vi "Teleop.vi"(8 "Begin Cluster":T1={"Left Drive Encoder"={"DevStatus"={"status"=FALSE, "code"=0, "source"=""}, "EncoderIndex"=enum."Invalid", "CounterIndex"=enum."Ctr 1", "DistancePerCount"=2.0, "Decoding Type"=enum."4x"}, "Right Drive Encoder"={"DevStatus"={"status"=FALSE, "code"=0, "source"=""}, "EncoderIndex"=enum."Invalid", "CounterIndex"=enum."Ctr 1", "DistancePerCount"=2.0, "Decoding Type"=enum."4x"}, "Elevator Encoder"={"DevStatus"={"status"=FALSE, "code"=0, "source"=""}, "EncoderIndex"=enum."Invalid", "CounterIndex"=enum."Ctr 1", "DistancePerCount"=2.0, "Decoding Type"=enum."4x"}, "Drive Shifter"={"DevStatus"={"status"=FALSE, "code"=0, "source"=""}, "Pneumatics Control Module"=0, "Forward Solenoid Channel"=enum."Invalid", "Reverse Solenoid Channel"=enum."Invalid"}, "Elevator Shifter"={"DevStatus"={"status"=FALSE, "code"=0, "source"=""}, "Pneumatics Control Module"=0, "Forward Solenoid Channel"=enum."Invalid", "Reverse Solenoid Channel"=enum."Invalid"}, "Elevator Brake"={"DevStatus"={"status"=FALSE, "code"=0, "source"=""}, "Pneumatics Control Module"=0, "Forward Solenoid Channel"=enum."Invalid", "Reverse Solenoid Channel"=enum."Invalid"}, "Intake Clamp"={"DevStatus"={"status"=FALSE, "code"=0, "source"=""}, "Pneumatics Control Module"=0, "Forward Solenoid Channel"=enum."Invalid", "Reverse Solenoid Channel"=enum."Invalid"}, "Intake Hinge"={"DevStatus"={"status"=FALSE, "code"=0, "source"=""}, "Pneumatics Control Module"=0, "Forward Solenoid Channel"=enum."Invalid", "Reverse Solenoid Channel"=enum."Invalid"}, "Pot Left"={"DevStatus"={"status"=FALSE, "code"=0, "source"=""}, "Analog Channel"=enum."Invalid", "Invert Output"=FALSE}, "Pot Right"={"DevStatus"={"status"=FALSE, "code"=0, "source"=""}, "Analog Channel"=enum."Invalid", "Invert Output"=FALSE}, "Gyro"={"DevStatus"={"status"=FALSE, "code"=0, "source"=""}, "Analog Channel"=enum."AI 1", "Gain (VoltsPerDegree/Second)"=0.0, "Gyro Type"=enum."Analog", "Handle"=0, "SPI Bus"=enum."Invalid", "Device Found"=FALSE, "Sample Rate"=1.0, "Calibrate On Open"=FALSE, "Offset"=0.0}, "Drive Motors"={"DevStatus"={"status"=FALSE, "code"=0, "source"=""}, "Motors[]"=[], "Square Inputs"=FALSE, "Max Output"=1.0}, "Elevator Master"={"DeviceStatus"={"status"=FALSE, "code"=0, "source"=""}, "Type"=enum."PWM", "PWM"={"PWM Channel"=enum."Invalid", "DeadBand"={"Name"="", "maxPositivePwm"=0, "minPositivePwm"=0, "centerPwm"=0, "maxNegativePwm"=0, "minNegativePwm"=0, "angularRange"=0}}, "CAN"={"Device Number"=0, "SetOutput VI Ref"=variant(refnum<vi> refnum), "GetOutput VI Ref"=variant(refnum<vi> refnum), "Enable VI Ref"=variant(refnum<vi> refnum), "Disable VI Ref"=variant(refnum<vi> refnum), "Data"=variant}, "Invert"=FALSE, "DIO PWM"={"PWM \"Enable\" Channel"=enum."Invalid", "DIOChannel"=enum."Invalid", "PWM Rate"=0.0}}, "Intake Left"={"DeviceStatus"={"status"=FALSE, "code"=0, "source"=""}, "Type"=enum."PWM", "PWM"={"PWM Channel"=enum."Invalid", "DeadBand"={"Name"="", "maxPositivePwm"=0, "minPositivePwm"=0, "centerPwm"=0, "maxNegativePwm"=0, "minNegativePwm"=0, "angularRange"=0}}, "CAN"={"Device Number"=0, "SetOutput VI Ref"=variant(refnum<vi> refnum), "GetOutput VI Ref"=variant(refnum<vi> refnum), "Enable VI Ref"=variant(refnum<vi> refnum), "Disable VI Ref"=variant(refnum<vi> refnum), "Data"=variant}, "Invert"=FALSE, "DIO PWM"={"PWM \"Enable\" Channel"=enum."Invalid", "DIOChannel"=enum."Invalid", "PWM Rate"=0.0}}, "Intake Right"={"DeviceStatus"={"status"=FALSE, "code"=0, "source"=""}, "Type"=enum."PWM", "PWM"={"PWM Channel"=enum."Invalid", "DeadBand"={"Name"="", "maxPositivePwm"=0, "minPositivePwm"=0, "centerPwm"=0, "maxNegativePwm"=0, "minNegativePwm"=0, "angularRange"=0}}, "CAN"={"Device Number"=0, "SetOutput VI Ref"=variant(refnum<vi> refnum), "GetOutput VI Ref"=variant(refnum<vi> refnum), "Enable VI Ref"=variant(refnum<vi> refnum), "Disable VI Ref"=variant(refnum<vi> refnum), "Data"=variant}, "Invert"=FALSE, "DIO PWM"={"PWM \"Enable\" Channel"=enum."Invalid", "DIOChannel"=enum."Invalid", "PWM Rate"=0.0}}, "Linear Actuator Left"={"DeviceStatus"={"status"=FALSE, "code"=0, "source"=""}, "Type"=enum."PWM", "PWM"={"PWM Channel"=enum."Invalid", "DeadBand"={"Name"="", "maxPositivePwm"=0, "minPositivePwm"=0, "centerPwm"=0, "maxNegativePwm"=0, "minNegativePwm"=0, "angularRange"=0}}, "CAN"={"Device Number"=0, "SetOutput VI Ref"=variant(refnum<vi> refnum), "GetOutput VI Ref"=variant(refnum<vi> refnum), "Enable VI Ref"=variant(refnum<vi> refnum), "Disable VI Ref"=variant(refnum<vi> refnum), "Data"=variant}, "Invert"=FALSE, "DIO PWM"={"PWM \"Enable\" Channel"=enum."Invalid", "DIOChannel"=enum."Invalid", "PWM Rate"=0.0}}, "Linear Actuator Right"={"DeviceStatus"={"status"=FALSE, "code"=0, "source"=""}, "Type"=enum."PWM", "PWM"={"PWM Channel"=enum."Invalid", "DeadBand"={"Name"="", "maxPositivePwm"=0, "minPositivePwm"=0, "centerPwm"=0, "maxNegativePwm"=0, "minNegativePwm"=0, "angularRange"=0}}, "CAN"={"Device Number"=0, "SetOutput VI Ref"=variant(refnum<vi> refnum), "GetOutput VI Ref"=variant(refnum<vi> refnum), "Enable VI Ref"=variant(refnum<vi> refnum), "Disable VI Ref"=variant(refnum<vi> refnum), "Data"=variant}, "Invert"=FALSE, "DIO PWM"={"PWM \"Enable\" Channel"=enum."Invalid", "DIOChannel"=enum."Invalid", "PWM Rate"=0.0}}, "X Joystick"={"Device"=enum."USB 1"}, "Y Joystick"={"Device"=enum."USB 1"}, "Controller"={"Device"=enum."USB 1"}, "775 Drive Motors"={"DevStatus"={"status"=FALSE, "code"=0, "source"=""}, "Motors[]"=[], "Square Inputs"=FALSE, "Max Output"=1.0}, "Intake Angle Encoder"={"DevStatus"={"status"=FALSE, "code"=0, "source"=""}, "EncoderIndex"=enum."Invalid", "CounterIndex"=enum."Ctr 1", "DistancePerCount"=2.0, "Decoding Type"=enum."4x"}, "Intake Angle"={"DeviceStatus"={"status"=FALSE, "code"=0, "source"=""}, "Type"=enum."PWM", "PWM"={"PWM Channel"=enum."Invalid", "DeadBand"={"Name"="", "maxPositivePwm"=0, "minPositivePwm"=0, "centerPwm"=0, "maxNegativePwm"=0, "minNegativePwm"=0, "angularRange"=0}}, "CAN"={"Device Number"=0, "SetOutput VI Ref"=variant(refnum<vi> refnum), "GetOutput VI Ref"=variant(refnum<vi> refnum), "Enable VI Ref"=variant(refnum<vi> refnum), "Disable VI Ref"=variant(refnum<vi> refnum), "Data"=variant}, "Invert"=FALSE, "DIO PWM"={"PWM \"Enable\" Channel"=enum."Invalid", "DIOChannel"=enum."Invalid", "PWM Rate"=0.0}}} {"Gyro"."Sample Rate" min=0.25 max=100.0 step=0.25}, 10 "Match Info":T20={"Autonomous Elapsed Seconds"=0.0, "TeleOp Elapsed Seconds"=0.0, "Disabled Elapsed Seconds"=0.0, "Visited Autonomous"=FALSE, "Visited TeleOp"=FALSE, "Visited Disabled"=FALSE, "Autonomous Settings"={"Autonomous Style"=enum."Independent", "VI Refnum"=refnum}}, 11 "Call Context":T21) -> ()   [LabVIEW 2017]
doc: "This VI is called for each TeleOp packet received from the DS where the robot is not disabled. It is often used to read from the joysticks and update I/O or to update setpoints for timed control loops. It should complete and return within 20 milliseconds or it may miss DS packets."
uses:
  <vilib>/Rock Robotics/WPI/DriverStation/WPI_DriverStationDerivedRobotMode.ctl
  <vilib>/Rock Robotics/WPI/DriverStation/WPI_DriverStationMatch Info.ctl
  Begin Cluster.ctl
  <vilib>/Rock Robotics/WPI/Encoder/WPI_EncoderDevRef.ctl
  <vilib>/Rock Robotics/SystemInterfaces/Encoder/FPGA_EncoderIdx.ctl
  <vilib>/Rock Robotics/SystemInterfaces/Counter/FPGA_CounterCtrSystemIndex.ctl
  <vilib>/Rock Robotics/WPI/Encoder/WPI_EncoderType.ctl
  <vilib>/Rock Robotics/WPI/Solenoid/WPI_SolenoidDevRef.ctl
  <vilib>/Rock Robotics/WPI/Solenoid/WPI_SolenoidChannel.ctl
  <vilib>/Rock Robotics/WPI/Potentiometer/WPI_PotentiometerDevRef.ctl
  <vilib>/Rock Robotics/SystemInterfaces/AI/FPGA_AIChannel.ctl
  <vilib>/Rock Robotics/WPI/Gyro/WPI_GyroDevRef.ctl
  <vilib>/Rock Robotics/SystemInterfaces/spilib/spi_bus.ctl
  <vilib>/Rock Robotics/WPI/RobotDrive/WPI_RobotDriveDevRef.ctl
  <vilib>/Rock Robotics/WPI/MotorControl/WPI_MotorControlDeviceRef.ctl
  <vilib>/Rock Robotics/WPI/MotorControl/WPI_MotorControlType.ctl
  <vilib>/Rock Robotics/SystemInterfaces/DIO/FPGA_DIOPWMChannel.ctl
  <vilib>/Rock Robotics/WPI/PWM/WPI_PWMDeadband.ctl
  <vilib>/Rock Robotics/SystemInterfaces/DIO/FPGA_DIOChannel.ctl
  <vilib>/Rock Robotics/WPI/Joystick/WPI_JoystickDevRef.ctl
  <vilib>/Rock Robotics/WPI/Joystick/WPI_JoystickDeviceEnum.ctl
  <vilib>/Rock Robotics/WPI/RobotDrive/WPI_RobotDriveArcadeDrive_Standard(NoSaturation).vi
  Global Variables.vi
panel:
  in  "Drive State":bool
  in  "Elevator State":bool
  # "Analog"
  # "XRS"
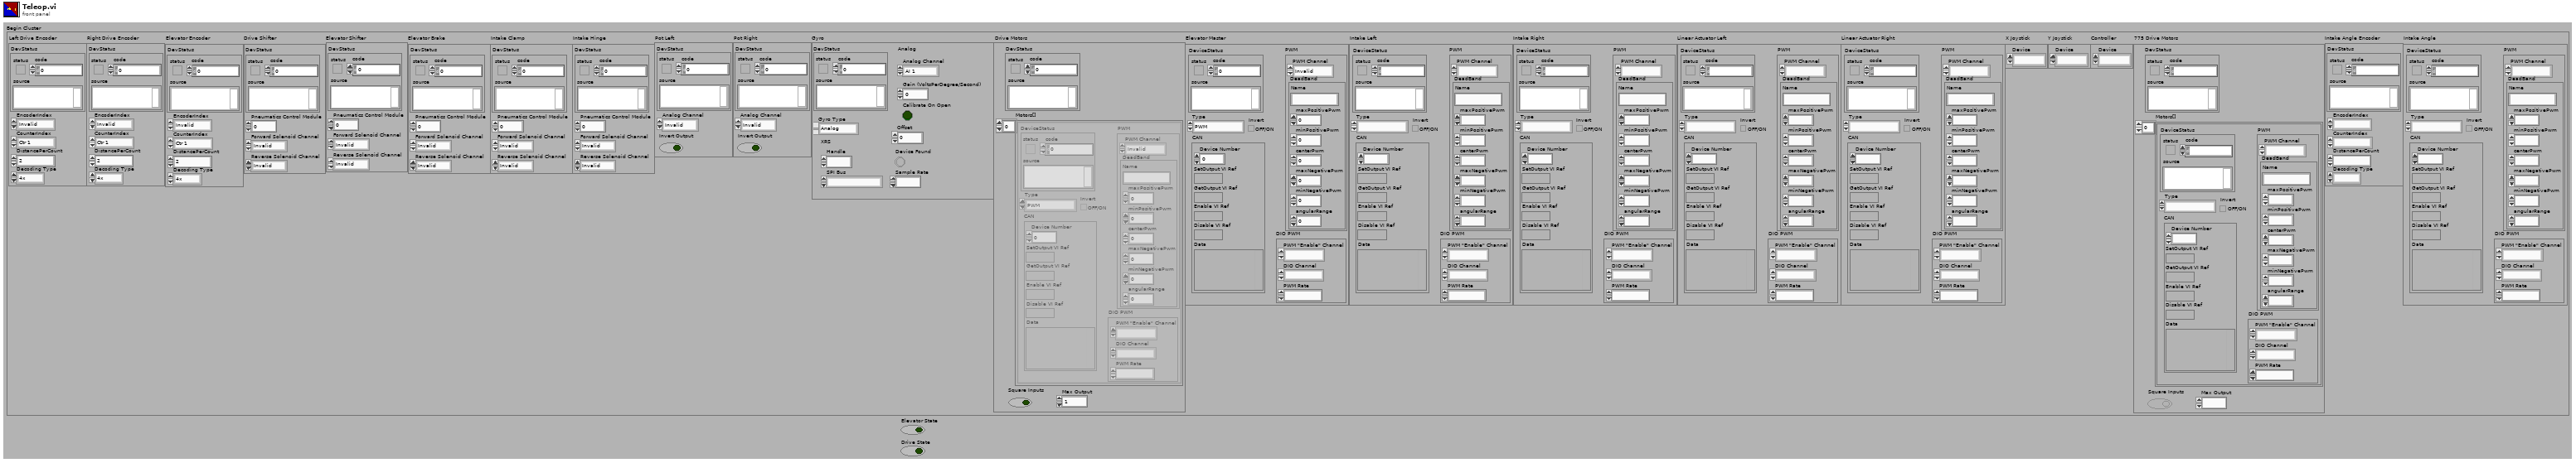
[diagram p1: front panel]
types:
  T1 = typedef "Begin Cluster.ctl" = cluster{"Left Drive Encoder":T2, "Right Drive Encoder":T2, "Elevator Encoder":T2, "Drive Shifter":T6, "Elevator Shifter":T6, "Elevator Brake":T6, "Intake Clamp":T6, "Intake Hinge":T6, "Pot Left":T8, "Pot Right":T8, "Gyro":T10, "Drive Motors":T12, "Elevator Master":T13, "Intake Left":T13, "Intake Right":T13, "Linear Actuator Left":T13, "Linear Actuator Right":T13, "X Joystick":T18, "Y Joystick":T18, "Controller":T18, "775 Drive Motors":T12, "Intake Angle Encoder":T2, "Intake Angle":T13}
  T2 = typedef "WPI_EncoderDevRef.ctl" = cluster{"DevStatus":errorcluster, "EncoderIndex":T3, "CounterIndex":T4, "DistancePerCount":dbl, "Decoding Type":T5}
  T3 = typedef "FPGA_EncoderIdx.ctl" = enum8{"Enc 0", "Enc 1", "Enc 2", "Enc 3", "Enc 4", "Enc 5", "Enc 6", "Enc 7", "Invalid"}
  T4 = typedef "FPGA_CounterCtrSystemIndex.ctl" = enum8{"Ctr 0", "Ctr 1", "Ctr 2", "Ctr 3", "Ctr 4", "Ctr 5", "Ctr 6", "Ctr 7", "Invalid"}
  T5 = typedef "WPI_EncoderType.ctl" = enum16{"1x", "2x", "4x"}
  T6 = typedef "WPI_SolenoidDevRef.ctl" = cluster{"DevStatus":errorcluster, "Pneumatics Control Module":u8, "Forward Solenoid Channel":T7, "Reverse Solenoid Channel":T7}
  T7 = typedef "WPI_SolenoidChannel.ctl" = enum8{"Solenoid 0", "Solenoid 1", "Solenoid 2", "Solenoid 3", "Solenoid 4", "Solenoid 5", "Solenoid 6", "Solenoid 7", "Invalid"}
  T8 = typedef "WPI_PotentiometerDevRef.ctl" = cluster{"DevStatus":errorcluster, "Analog Channel":T9, "Invert Output":bool}
  T9 = typedef "FPGA_AIChannel.ctl" = enum8{"AI 0", "AI 1", "AI 2", "AI 3", "AI MXP 0", "AI MXP 1", "AI MXP 2", "AI MXP 3", "Invalid"}
  T10 = typedef "WPI_GyroDevRef.ctl" = cluster{"DevStatus":errorcluster, "Analog Channel":T9, "Gain (VoltsPerDegree/Second)":dbl, "Gyro Type":enum16{"Analog", "XRS450"}, "Handle":i32, "SPI Bus":T11, "Device Found":bool, "Sample Rate":dbl, "Calibrate On Open":bool, "Offset":dbl}
  T11 = typedef "spi_bus.ctl" = enum16{"SPI On-Board, CS0", "SPI On-Board, CS1", "SPI On-Board, CS2", "SPI On-Board, CS3", "SPI MXP", "Invalid"}
  T12 = typedef "WPI_RobotDriveDevRef.ctl" = cluster{"DevStatus":errorcluster, "Motors[]":T13[], "Square Inputs":bool, "Max Output":dbl}
  T13 = typedef "WPI_MotorControlDeviceRef.ctl" = cluster{"DeviceStatus":errorcluster, "Type":T14, "PWM":cluster{"PWM Channel":T15, "DeadBand":T16}, "CAN":cluster{"Device Number":u8, "SetOutput VI Ref":variant, "GetOutput VI Ref":variant, "Enable VI Ref":variant, "Disable VI Ref":variant, "Data":variant}, "Invert":bool, "DIO PWM":cluster{"PWM \"Enable\" Channel":T15, "DIOChannel":T17, "PWM Rate":dbl}}
  T14 = typedef "WPI_MotorControlType.ctl" = enum16{"PWM", "CAN", "DIO PWM"}
  T15 = typedef "FPGA_DIOPWMChannel.ctl" = enum8{"PWM 0", "PWM 1", "PWM 2", "PWM 3", "PWM 4", "PWM 5", "PWM 6", "PWM 7", "PWM 8", "PWM 9", "PWM MXP 0", "PWM MXP 1", "PWM MXP 2", "PWM MXP 3", "PWM MXP 4", "PWM MXP 5", "PWM MXP 6", "PWM MXP 7", "PWM MXP 8", "PWM MXP 9", "Invalid"}
  T16 = typedef "WPI_PWMDeadband.ctl" = cluster{"Name":string, "maxPositivePwm":i32, "minPositivePwm":i32, "centerPwm":i32, "maxNegativePwm":i32, "minNegativePwm":i32, "angularRange":u16}
  T17 = typedef "FPGA_DIOChannel.ctl" = enum8{"DIO 0", "DIO 1", "DIO 2", "DIO 3", "DIO 4", "DIO 5", "DIO 6", "DIO 7", "DIO 8", "DIO 9", "DIO MXP 0", "DIO MXP 1", "DIO MXP 2", "DIO MXP 3", "DIO MXP 4", "DIO MXP 5", "DIO MXP 6", "DIO MXP 7", "DIO MXP 8", "DIO MXP 9", "DIO MXP 10", "DIO MXP 11", "DIO MXP 12", "DIO MXP 13", "DIO MXP 14", "DIO MXP 15", "SPI Port CS1", "SPI Port CS2", "SPI Port CS3", "SPI Port MISO", "SPI Port MOSI", "Invalid"}
  T18 = typedef "WPI_JoystickDevRef.ctl" = cluster{"Device":T19}
  T19 = typedef "WPI_JoystickDeviceEnum.ctl" = enum16{"USB 0", "USB 1", "USB 2", "USB 3", "USB 4", "USB 5"}
  T20 = typedef "WPI_DriverStationMatch Info.ctl" = cluster{"Autonomous Elapsed Seconds":dbl, "TeleOp Elapsed Seconds":dbl, "Disabled Elapsed Seconds":dbl, "Visited Autonomous":bool, "Visited TeleOp":bool, "Visited Disabled":bool, "Autonomous Settings":cluster{"Autonomous Style":enum16{"Iterative", "Independent"}, "VI Refnum":refnum<vi>}}
  T21 = typedef "WPI_DriverStationDerivedRobotMode.ctl" = enum16{"Init", "Execute", "Stop"}
  T22 = enum16{"Idle", "Portal", "Subtract", "Add", "Straight Up"}
  T23 = enum16{"Idle", "Ground", "Portal", "Switch", "Scale", "Cube Down", "Cube Up", "Add Down", "Add Up"}
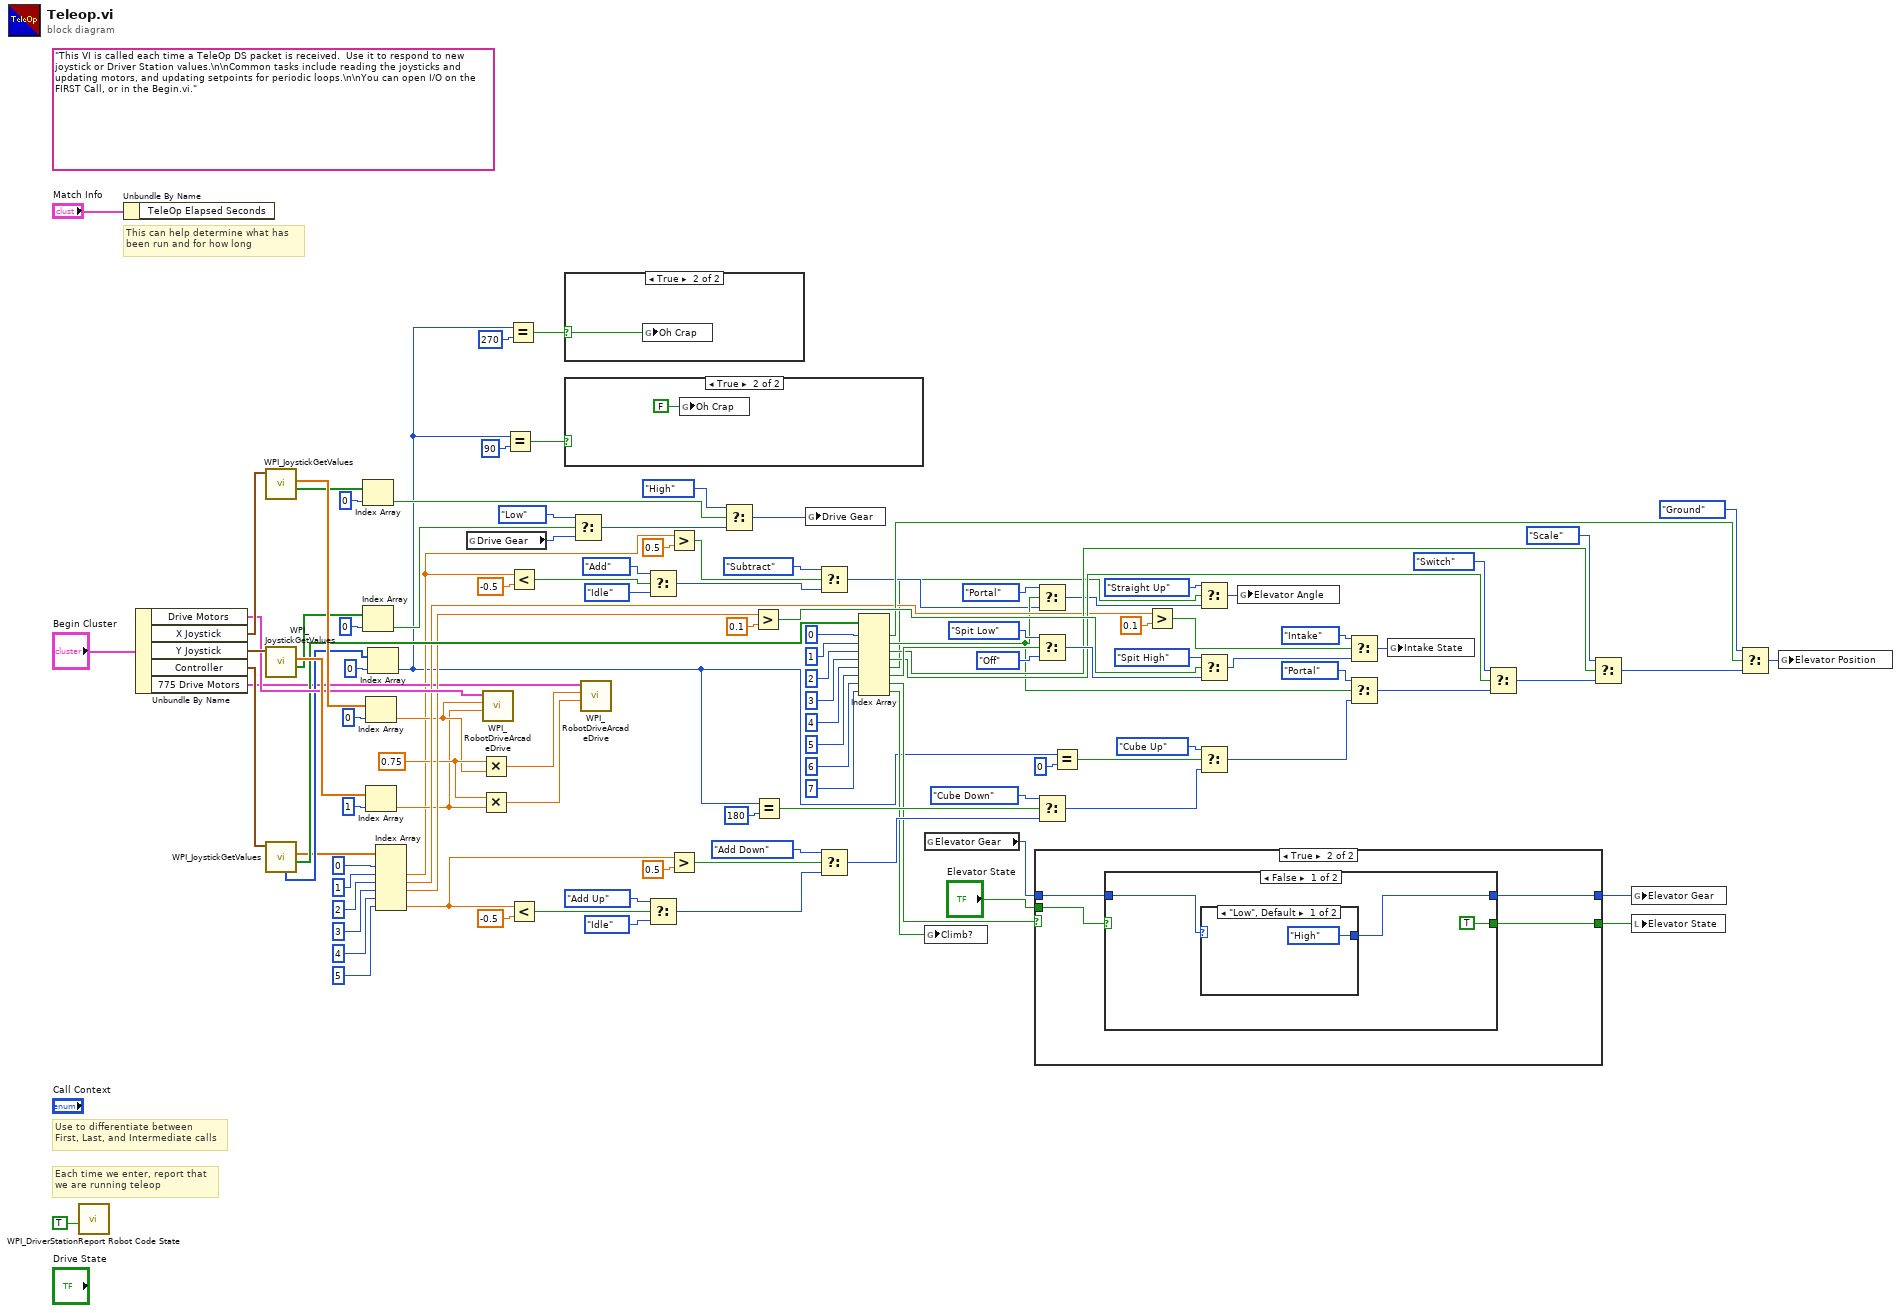
[diagram p0: block diagram]
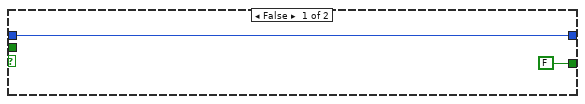
[diagram p4: hidden frame]
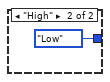
[diagram p5: hidden frame]
diagram:
  w37 = 0.75 ("x")
  (unwired) "This VI is called each time a TeleOp DS packet is received.  Use it to respond to new joystick or Driver Station values.\n\nCommon tasks include reading the joysticks and updating motors, and updating setpoints for periodic loops.\n\nYou can open I/O on the FIRST Call, or in the Begin.vi."
  # "Each time we enter, report that\nwe are running teleop"
  # "Use to differentiate between\nFirst, Last, and Intermediate calls"
  # "This can help determine what has\nbeen run and for how long"
  n1 = call <vilib>:"WPI_DriverStationReport Robot Code State.vi"("TeleOp"=TRUE ("Autonomous")) -> ()  [unwired: 10 in, 1 out]
  n2 = Unbundle By Name("Match Info") -> ()  [unwired: 1 out]
  n3 = Unbundle By Name("Begin Cluster") -> ("Drive Motors"=w107:T12, "X Joystick"=w113:T18, "Y Joystick"=w112:T18, "Controller"=w106:T18, "775 Drive Motors"=w32:T12)
  n4 = call <vilib>:"WPI_JoystickGetValues.vi"("JoystickDevRef"=w113) -> ("Buttons"=w50:bool[], "Axes"=w111:dbl[])  [unwired: 6 in, 3 out]
  n5 = call <vilib>:"WPI_JoystickGetValues.vi"("JoystickDevRef"=w112) -> ("Buttons"=w49:bool[], "Axes"=w110:dbl[])  [unwired: 6 in, 3 out]
  n6 = call <vilib>:"WPI_JoystickGetValues.vi"("JoystickDevRef"=w106) -> ("Buttons"=w105:bool[], "Axes"=w95:dbl[], "POVs"=w96:i16[])  [unwired: 6 in, 2 out]
  n7 = Index Array(array=w50, index=0) -> (element=w41:bool)
  n8 = Index Array(array=w49, index=0) -> (element=w40:bool)
  n9 = Index Array(array=w111, index=0) -> (element=w36:dbl)
  n10 = Index Array(array=w110, index=1) -> (element=w35:dbl)
  n11 = Index Array(array=w96, index=0) -> (element=w2:i16)
  n12 = Index Array(array=w95, index #1=0 ("index"), index #2=1 ("index"), index #3=2 ("index"), index #4=3 ("index"), index #5=4 ("index"), index #6=5 ("index")) -> (element #2=w8:dbl, element #3=w38:dbl, element #4=w39:dbl, element #6=w67:dbl)  [unwired: 2 out]
  n13 = global read "Global Variables.vi" "Drive Gear"() -> (w45:enum16{"Low", "High"})
  n14 = Multiply(x=w37, y=w36) -> (x*y=w33:dbl)
  n15 = Multiply(x=w37, y=w35) -> (x*y=w34:dbl)
  n16 = call-poly <vilib>:"WPI_RobotDriveArcadeDrive.vi"("Y axis value"=w35, "X axis value"=w36, "RobotDriveDevRef"=w107) -> ()  [unwired: 6 in, 3 out]
  n17 = Equal?(x=w2, y=i16 90) -> (x = y?=w1:bool)
  n18 = Equal?(x=w2, y=i16 270) -> (x = y?=w4:bool)
  n19 = Less?(x=w8, y=-0.5) -> (x < y?=w18:bool)
  n20 = Less?(x=w67, y=-0.5) -> (x < y?=w64:bool)
  n21 = case shown="True" w4 {
    selector: w4 -> [_ w117]
    frame False {
    }
    frame True {
      n22 = global write "Global Variables.vi" "Oh Crap"(w117) -> ()
    }
  }
  n23 = case shown="True" w1 {
    frame False {
    }
    frame True {
      n24 = global write "Global Variables.vi" "Oh Crap"(FALSE ("Oh Crap")) -> ()
    }
  }
  n25 = Select(t=enum16{"Low", "High"}."Low", s=w40, f=w45) -> (s? t:f=w46:enum16{"Low", "High"})
  n26 = call-poly <vilib>:"WPI_RobotDriveArcadeDrive.vi"("Y axis value"=w34, "X axis value"=w33, "RobotDriveDevRef"=w32) -> ()  [unwired: 6 in, 3 out]
  n27 = Select(t=T22."Add", s=w18, f=T22."Idle" ("Elevator Angle")) -> (s? t:f=w17:T22)
  n28 = Select(t=T23."Add Up", s=w64, f=T23."Idle") -> (s? t:f=w76:T23)
  n29 = Greater?(x=w8, y=0.5) -> (0:w19:bool)
  n30 = Greater?(x=w67, y=0.5) -> (0:w63:bool)
  n31 = Select(t=enum16{"Low", "High"}."High", s=w41, f=w46) -> (s? t:f=w44:enum16{"Low", "High"})
  n32 = Greater?(x=w39, y=0.1) -> (0:w85:bool)
  n33 = Equal?(x=w2, y=i16 180) -> (x = y?=w56:bool)
  n34 = global write "Global Variables.vi" "Drive Gear"(w44) -> ()
  n35 = Select(t=T22."Subtract", s=w19, f=w17) -> (s? t:f=w16:T22)
  n36 = Select(t=T23."Add Down", s=w63, f=w76) -> (s? t:f=w75:T23)
  n37 = Index Array(array=w105, index #1=0 ("index"), index #2=1 ("index"), index #3=2 ("index"), index #4=3 ("index"), index #5=4 ("index"), index #6=5 ("index"), index #7=6 ("index"), index #8=7 ("index")) -> (element #1=w70:bool, element #2=w22:bool, element #3=w62:bool, element #4=w61:bool, element #5=w7:bool, element #6=w83:bool, element #7=w51:bool, element #8=w6:bool)
  n38 = global read "Global Variables.vi" "Elevator Gear"() -> (w55:enum16{"Low", "High"})
  n39 = global write "Global Variables.vi" "Climb?"(w6) -> ()
  n40 = case shown="True" w51 {
    tunnel: [FALSE w124] -> w53
    tunnel: w55 -> [w119 w123]
    tunnel: [w119 w122] -> w54
    tunnel: "Elevator State" -> [_ w121]
    frame False {
    }
    frame True {
      n41 = case shown="False" w121 {
        selector: w121 -> [_ w131]
        tunnel: [TRUE w131] -> w124
        tunnel: w123 -> [w126 w130]
        tunnel: [w125 w130] -> w122
        frame False {
          n42 = case shown="\"Low\", Default" w126 {
            tunnel: [enum16{"Low", "High"}."High" ("Elevator Gear") enum16{"Low", "High"}."Low" ("Elevator Gear")] -> w125
            frame "Low", Default {
            }
            frame "High" {
            }
          }
        }
        frame True {
        }
      }
    }
  }
  n43 = Select(t=T22."Portal", s=w22, f=w16) -> (s? t:f=w15:T22)
  n44 = Select(t=enum16{"Off", "Intake", "Spit Low", "Spit High"}."Spit Low" ("Intake State"), s=w83, f=enum16{"Off", "Intake", "Spit Low", "Spit High"}."Off" ("Intake State")) -> (s? t:f=w77:enum16{"Off", "Intake", "Spit Low", "Spit High"})
  n45 = Select(t=T23."Cube Down", s=w56, f=w75) -> (s? t:f=w74:T23)
  n46 = Equal?(x=w2, y=i16 0) -> (x = y?=w58:bool)
  n47 = Greater?(x=w38, y=0.1) -> (0:w86:bool)
  n48 = Select(t=T22."Straight Up", s=w7, f=w15) -> (s? t:f=w9:T22)
  n49 = Select(t=enum16{"Off", "Intake", "Spit Low", "Spit High"}."Spit High" ("Intake State"), s=w85, f=w77) -> (s? t:f=w84:enum16{"Off", "Intake", "Spit Low", "Spit High"})
  n50 = Select(t=T23."Cube Up", s=w58, f=w74) -> (s? t:f=w73:T23)
  n51 = global write "Global Variables.vi" "Elevator Angle"(w9) -> ()
  n52 = Select(t=enum16{"Off", "Intake", "Spit Low", "Spit High"}."Intake" ("Intake State"), s=w86, f=w84) -> (s? t:f=w78:enum16{"Off", "Intake", "Spit Low", "Spit High"})
  n53 = Select(t=T23."Portal", s=w22, f=w73) -> (s? t:f=w72:T23)
  n54 = global write "Global Variables.vi" "Intake State"(w78) -> ()
  n55 = Select(t=T23."Switch", s=w61, f=w72) -> (s? t:f=w71:T23)
  n56 = Select(t=T23."Scale", s=w62, f=w71) -> (s? t:f=w69:T23)
  n57 = global write "Global Variables.vi" "Elevator Gear"(w54) -> ()
  n58 = local write "Elevator State"(w53) -> ()
  n59 = Select(t=T23."Ground", s=w70, f=w69) -> (s? t:f=w68:T23)
  n60 = global write "Global Variables.vi" "Elevator Position"(w68) -> ()
